vi "Main Low-T Experiments.vi"() -> ()   [LabVIEW 2012]
uses:
  Global Vars.vi
  Channels.vi
  States.ctl
  <vilib>/DAQmx/read.llb/DAQmx Read (Counter U32 1Chan 1Samp).vi
  <vilib>/DAQmx/create/channels.llb/DAQmx Create Channel (CI-Count Edges).vi
  Strict Type Def - Scan Parameters Cluster.ctl
  Rabi Window Parameters.ctl
  ESR Window Parameters.ctl
  Strict Type Def - Optimize Parameters Cluster.ctl
  Spin Echo Window Parameters.ctl
  low-T/Spectrum Window Parameters.ctl
  low-T/Stability Window Parameters.ctl
  Window Parameters-CPMG.ctl
  SaveContrastOptions.ctl
  Window Parameters-XY4.ctl
panel:
  in  "Program":T1(tab)
  in  "Continuous":bool
  in  "Green Laser (low-T)":bool caption="Scan"
  in  "Microwave":bool caption="Scan"
  in  "Green Laser":bool caption="Scan"
  out "Counts Intensity Graph":i32[][](graph)
  in  "Scan Parameters":T2={"X Max"=1.0, "X Min"=-1.0, "X Step"=0.01, "Y Max"=1.5, "Y Min"=-1.5, "Y Step"=0.01, "Dwell Time (ms) "=1} {"Dwell Time (ms)" min=0; "Y Step" min=0.0; "X Step" min=0.0}
  in  "Optimize":bool
  in  "Scan":bool
  in  "Count":bool caption="Optimize"
  out "Counts Chart":u32(graph)
  out "Counts/s":i32
  in  "Optimize Parameters":T3={"Volt Step"={"X"=0.01, "Y"=0.01, "Z"=0.0}, "Num Iterations"=5, "Dwell Time (ms)"=10, "Volts Range"={"X"=0.1, "Y"=0.1, "Z"=0.0}, "Method"={"X"=enum."Max", "Y"=enum."Max"}} {"Volts Range"."Z" min=0.0; "Volts Range"."Y" min=0.0; "Volts Range"."X" min=0.0; "Dwell Time (ms)" min=0; "Num Iterations" min=1 step=1; "Volt Step"."Z" min=0.0; "Volt Step"."Y" min=1e-06; "Volt Step"."X" min=1e-06}
  in  "ESR":bool caption="Scan"
  in  "ESR spectrum spreadsheet":path=path "C:/experiment/data/may_15_2012/SIL1_NV1_pippin_uW_off"
  in  "Save ESR spectrum data":bool
  in  "ESR spectrum graph":path=path "C:/experiment/data/may_15_2012/SIL1_NV1_pippin_uW_off"
  in  "Save ESR spectrum graph":bool
  out "Avg ESR spectrum":cluster{"Y":dbl[], "Y":dbl[]}[](graph)
  out "Counts vs. frequency":i32[][](graph)
  in  "# freq points":i32=61
  in  "MW start freq (GHz)":dbl=2.84
  in  "MW stop freq (GHz)":dbl=2.9
  in  "# scans before track":i32=10
  in  "#scan iterations":i32=5
  in  "ESR Parameters":T4={"Window 1 time (s)"=0.012, "Window 2 time (s)"=5e-06, "Window 3 time (s) "=0.02, "Window 4 time (s)"=5e-07, "Window 4 channels"=[TRUE, FALSE, FALSE, TRUE], "Window 3 channels"=[TRUE, FALSE, TRUE, TRUE], "Window 2 channels"=[TRUE, FALSE, FALSE, TRUE], "Window 1 channels"=[TRUE, TRUE, FALSE, TRUE], "Path to ESR Burner"=path "C:/Users/Loncar/Desktop/ESR VIs - Srujan/Sam Kim/PB/ESRFreq.exe"}
  in  "Save Rabi Contrast Options":T5={"Save contrast graph"=FALSE, "Path for contrast graph"=path "C:/experiment/data/may_15_2012/SIL1_NV1_pippin_uW_off", "Save contrast data"=FALSE, "Path for contrast data"=path "C:/experiment/data/may_15_2012/SIL1_NV1_pippin_uW_off"}
  in  "# scan iterations":i32
  in  "Rabi Parameters":T6={"Window 1 time (s)"=3e-06, "Window 2 time (s)"=5e-06, "Window 3 min time (s) "=0.0, "Window 3 max time (s)"=0.0, "Window 4 time (s)"=7.5e-07, "Window 5 time (s)"=2e-07, "Window 6 time (s)"=3e-06, "Window 7 time (s)"=2e-07, "Window 8 time (s)"=1e-07, "# samples before track"=0, "# time axis points"=0, "Window 1 active channels"=[FALSE, FALSE, FALSE, TRUE], "Window 2 active channels"=[], "Window 3 active channels"=[TRUE], "Window 4 active channels"=[FALSE, FALSE, FALSE, TRUE], "Window 5 active channels "=[FALSE, FALSE, TRUE, TRUE], "Window 6 active channels"=[FALSE, FALSE, FALSE, TRUE], "Window 7 active channels"=[FALSE, FALSE, TRUE, TRUE], "Window 8 active channels"=[], "Path to Rabi Burner"=path "C:/Users/Loncar/Desktop/ESR VIs - Srujan/Sam Kim/PB/RabiBurn.exe"}
  out "Rabi Normalized contrast":cluster{"Y":dbl[], "Y":dbl[]}[](graph)
  out "Reference counts":cluster{"Y":dbl[], "Y":dbl[]}[](graph)
  out "Readout counts":cluster{"Y":dbl[], "Y":dbl[]}[](graph)
  in  "Rabi":bool caption="Scan"
  in  "SpinEcho Save Options":T5={"Save contrast graph"=FALSE, "Path for contrast graph"=path "C:/experiment/data/may_15_2012/SIL1_NV1_pippin_uW_off", "Save contrast data"=FALSE, "Path for contrast data"=path "C:/experiment/data/may_15_2012/SIL1_NV1_pippin_uW_off"}
  in  "# SpinEcho scan iterations":i32=2
  in  "Spin Echo Parameters":T7={"Path to Spin Echo Burner"=path "C:/Users/Loncar/Desktop/ESR VIs - Srujan/Sam Kim/PB/SpinEchoBurn.exe", "Window 1 time (s)"=3e-06, "Window 1 active channels"=[FALSE, FALSE, FALSE, TRUE], "Window 10 time (s)"=3e-06, "Window 10 active channels"=[FALSE, FALSE, FALSE, TRUE], "# samples"=0, "Window 2 time (s)"=5e-06, "Window 2 active channels"=[], "Window 4 min time (s) "=0.0, "Window 4 active channels"=[FALSE], "Window 8 time (s)"=7.5e-07, "Window 8 active channels"=[FALSE, FALSE, FALSE, TRUE], "Window 9 time (s)"=2e-07, "Window 9 active channels "=[FALSE, FALSE, TRUE, TRUE], "# time axis points"=0, "Window 11 time (s)"=2e-07, "Window 11 active channels"=[FALSE, FALSE, TRUE, TRUE], "Window 12 time (s)"=1e-07, "Window 12 active channels"=[], "Window 4 max time (s)"=0.0, "Window 3 time (s)"=5e-06, "Window 5 time (s)"=5e-06, "Window 3 active channels"=[TRUE, FALSE, FALSE, FALSE], "Window 5 active channels"=[TRUE, FALSE, FALSE, FALSE], "Window 7 time (s)"=5e-06, "Window 7 active channels"=[TRUE, FALSE, FALSE, FALSE]}
  out "Spin Echo contrast":cluster{"Y":dbl[], "Y":dbl[]}[](graph)
  out "Spin Echo Reference":cluster{"Y":dbl[], "Y":dbl[]}[](graph)
  out "SpinEcho Readout":cluster{"Y":dbl[], "Y":dbl[]}[](graph)
  in  "Spin Echo":bool caption="Scan"
  in  "Spectrum":bool caption="Scan"
  out "Average counts":picture
  in  "Path for avg spectrum spreadsheet":path=path "C:/experiment/data/may_15_2012/SIL1_NV1_pippin_uW_off"
  in  "Save avg counts data":bool
  in  "Path for avg spectrum graph":path=path "C:/experiment/data/may_15_2012/SIL1_NV1_pippin_uW_off"
  in  "Save avg spectrum graph":bool
  in  "Save 2D counts array":bool
  in  "Path for 2D counts spreadsheet":path=path "C:/experiment/data/may_15_2012/SIL1_NV1_pippin_uW_off"
  in  "Path for intensity graph":path=path "C:/experiment/data/may_15_2012/SIL1_NV1_pippin_uW_off"
  in  "Save intensity graph":bool
  out "Counts vs. laser voltage":u32[][](graph)
  in  "# V steps":dbl
  in  "V max":dbl=0.3
  in  "V min":dbl=-0.3
  in  "# scans before tracking":i32
  in  "# Spectrum Scan Iterations":i32
  in  "Spectrum Parameters":T8={"Window 1 time (s)"=2e-05, "Window 2 time (s)"=1e-06, "Window 3 time (s) "=5e-08, "Window 4 time (s)"=2e-06, "Path to SpectrumBurn"=path "C:/Users/Loncar/Desktop/ESR VIs - Srujan/Sam Kim/PB/ESRFreq.exe", "Window 5 time (s)"=1e-07, "Window 6 time (s)"=5e-08, "Window 1 active channels"=[FALSE, TRUE], "Window 2 active channels"=[], "Window 3 active channels "=[FALSE, FALSE, TRUE], "Window 4 active channels"=[TRUE, FALSE, TRUE], "Window 5 active channels"=[FALSE, FALSE, TRUE], "Window 6 active channels"=[]}
  in  "Stability":bool caption="Scan"
  in  "Num Scan Iterations":i32
  in  "# V steps":dbl
  in  "V max":dbl=0.3
  in  "V min":dbl=-0.3
  in  "# scans before tracking":i32
  in  "Stability Parameters":T9={"Window 1 time (s)"=2e-05, "Window 2 time (s)"=1e-06, "Window 3 time (s) "=5e-08, "Window 4 time (s)"=2e-06, "Window 5 time (s)"=1e-07, "Window 6 time (s)"=5e-08, "Path to StabilityBurn"=path "C:/Users/Loncar/Desktop/ESR VIs - Srujan/Sam Kim/PB/StabilityBurn.exe", "Window 1 active channels"=[FALSE, TRUE], "Window 2 active channels"=[], "Window 3 active channels "=[FALSE, FALSE, TRUE], "Window 4 active channels"=[TRUE, FALSE, TRUE], "Window 5 active channels"=[FALSE, FALSE, TRUE], "Window 6 active channels"=[]}
  out "Counts vs. laser voltage":u32[][](graph)
  in  "Save intensity graph":bool
  in  "Path for intensity graph":path=path "C:/experiment/data/may_15_2012/SIL1_NV1_pippin_uW_off"
  in  "Path for 2D counts spreadsheet":path=path "C:/experiment/data/may_15_2012/SIL1_NV1_pippin_uW_off"
  in  "Save 2D counts array":bool
  in  "Save avg stability graph":bool
  in  "Path for avg stability graph":path=path "C:/experiment/data/may_15_2012/SIL1_NV1_pippin_uW_off"
  in  "Save avg counts data":bool
  in  "Path for avg spectrum spreadsheet":path=path "C:/experiment/data/may_15_2012/SIL1_NV1_pippin_uW_off"
  out "Average counts":picture
  in  "Save CPMG Contrast Options":T5={"Save contrast graph"=FALSE, "Path for contrast graph"=path "C:/experiment/data/may_15_2012/SIL1_NV1_pippin_uW_off", "Save contrast data"=FALSE, "Path for contrast data"=path "C:/experiment/data/may_15_2012/SIL1_NV1_pippin_uW_off"}
  out "CPMG contrast":cluster{"Y":dbl[], "Y":dbl[]}[](graph)
  out "CPMG Reference counts":cluster{"Y":dbl[], "Y":dbl[]}[](graph)
  out "CPMG Readout counts":cluster{"Y":dbl[], "Y":dbl[]}[](graph)
  in  "CPMG":bool caption="Scan"
  in  "# scan iterations":i32
  in  "CPMG Parameters":T10={"Path to CPMG Burner"=path "C:/Users/Loncar/Desktop/ESR VIs - Srujan/Sam Kim/PB/SpinEchoBurn.exe", "Window 1 time (s)"=3e-06, "Window 1 active channels"=[FALSE, FALSE, FALSE, TRUE], "Window 10 time (s)"=3e-06, "Window 10 active channels"=[FALSE, FALSE, FALSE, TRUE], "Window 2 time (s)"=0.0, "Window 2 active channels"=[], "Window 4 min time (s) "=0.0, "Window 4 active channels"=[FALSE], "Window 8 time (s)"=7.5e-07, "Window 8 active channels"=[FALSE, FALSE, FALSE, TRUE], "Window 9 time (s)"=2e-07, "Window 9 active channels "=[FALSE, FALSE, TRUE, TRUE], "# delay time points"=2, "Window 11 time (s)"=0.0, "Window 11 active channels"=[FALSE, FALSE, TRUE, TRUE], "Window 12 time (s)"=1e-07, "Window 12 active channels"=[], "Window 4 max time (s)"=0.0, "Window 3 time (s)"=0.0, "Window 5 time (s)"=5e-06, "Window 3 active channels"=[TRUE, FALSE, FALSE, FALSE], "Window 5 active channels"=[TRUE, FALSE, FALSE, FALSE], "# pi pulses"=1, "# samples before track"=0} {"# pi pulses" min=1; "# delay time points" min=2}
  in  "Save XY-4 Contrast Options":T5={"Save contrast graph"=FALSE, "Path for contrast graph"=path "C:/experiment/data/may_15_2012/SIL1_NV1_pippin_uW_off", "Save contrast data"=FALSE, "Path for contrast data"=path "C:/experiment/data/may_15_2012/SIL1_NV1_pippin_uW_off"}
  out "XY-4 Normalized contrast":cluster{"Y":dbl[], "Y":dbl[]}[](graph)
  out "XY-4 Reference counts":cluster{"Y":dbl[], "Y":dbl[]}[](graph)
  out "XY-4 Readout counts":cluster{"Y":dbl[], "Y":dbl[]}[](graph)
  in  "XY-4":bool caption="Scan"
  in  "# scan iterations":i32
  in  "XY-4 Parameters":T11={"Path to CPMG Burner"=path "C:/Users/Loncar/Desktop/ESR VIs - Srujan/Sam Kim/PB/SpinEchoBurn.exe", "Window 1 time (s)"=3e-06, "Window 1 active channels"=[FALSE, FALSE, FALSE, TRUE], "Window 10 time (s)"=3e-06, "Window 10 active channels"=[FALSE, FALSE, FALSE, TRUE], "Window 2 time (s)"=0.0, "Window 2 active channels"=[], "Window 4 min time (s) "=0.0, "Window 4 active channels"=[FALSE], "Window 8 time (s)"=7.5e-07, "Window 8 active channels"=[FALSE, FALSE, FALSE, TRUE], "Window 9 time (s)"=2e-07, "Window 9 active channels "=[FALSE, FALSE, TRUE, TRUE], "# time points"=2, "Window 11 time (s)"=0.0, "Window 11 active channels"=[FALSE, FALSE, TRUE, TRUE], "Window 12 time (s)"=1e-07, "Window 12 active channels"=[], "Window 4 max time (s)"=0.0, "Window 3 time (s)"=0.0, "Window 5 time (s)"=5e-06, "Window 3 active channels"=[TRUE, FALSE, FALSE, FALSE], "Window 5c active channels"=[TRUE, FALSE, FALSE, FALSE], "# pulse sequences"=1, "# samples before track"=0, "Window 5a active channels"=[TRUE, FALSE, FALSE, FALSE]} {"# pulse sequences" min=1; "# time points" min=2}
  in  "Laser voltage":tag="Dev1/ao2"
  in  "Counter(s)":tag="Dev1/ctr0"
  in  "X AO Channel":tag="Dev1/ao0"
  in  "Y AO Channel":tag="Dev1/ao1"
  in  "Sample clock line":tag="/Dev1/PFI9"
  in  "spinapi.dll":path=path "C:/SpinCore/SpinAPI/dll/spinapi64.dll"
  in  "HoldChannel.exe":path=path "C:/Users/Loncar/Desktop/ESR VIs - Srujan/Sam Kim/PB/HoldChannel.exe"
  # "Default PB connections:\nPB0 - MW switch\nPB3 - Green AOM\nDefault for low-T:\nPB1 - Green AOM"
  # "ESR spectrum measurement"
  # "Default PB connections:\nPB0 - MW switch\nPB1 - MW freq step\nPB2 - Counter sample clk\nPB3 - Green AOM"
  # "Pulse sequence parameters - Window durations and PB channel states"
  # "Green AOM, MW switch are always on!"
  # "(to spreadsheet)"
  # "MW freq step\ndwell time"
  # "MW freq step"
  # "Wait"
  # "Fluorescence\ncounting"
  # "Ctr sample clk"
  # "Wait"
  # "Rabi measurement"
  # "Default PB connections:\nPB0 - MW switch\nPB1 - unused\nPB2 - Counter sample clk\nPB3 - Green AOM"
  # "to spreadsheet"
  # "Initialization"
  # "Green AOM"
  # "Wait"
  # "All off"
  # "MW pulsing"
  # "MW"
  # "Wait"
  # "Green AOM"
  # "Green AOM,\ncounter sample clk"
  # "Readout"
  # "Repump"
  # "Green AOM"
  # "Green AOM,\ncounter sample clk"
  # "Reference"
  # "All off"
  # "Wait (nominal)"
  # "Spin Echo measurement"
  # "Default PB connections:\nPB0 - MW switch\nPB1 - unused\nPB2 - Counter sample clk\nPB3 - Green AOM"
  # "to spreadsheet"
  # "Green AOM"
  # "Initialization"
  # "All off"
  # "Wait"
  # "MW"
  # "MW pulse 1"
  # "All off"
  # "Free precession 1"
  # "max: ~350"
  # "MW pulse 2"
  # "MW"
  # "Free precession 2: Window 6"
  # "MW"
  # "MW pulse 1"
  # "Green AOM"
  # "Wait"
  # "Green AOM,\ncounter sample clk"
  # "Readout"
  # "Green AOM"
  # "Repump"
  # "Green AOM,\ncounter sample clk"
  # "Reference"
  # "Wait (nominal)"
  # "All off"
  # "(single shot) resonance fluorescence spectroscopy"
  # "Default PB connections:\nPB0 - Red AOM\nPB1 - Green AOM\nPB2 - Counter sample clk"
  # "(to spreadsheet)"
  # "(to spreadsheet)"
  # "Laser Set:"
  # "Spectral stability characterization"
  # "Default PB connections:\nPB0 - Red AOM\nPB1 - Green AOM\nPB2 - Counter sample clk"
  # "(to spreadsheet)"
  # "Laser Set:"
  # "(to spreadsheet)"
  # "CPMG measurement"
  # "Default PB connections:\nPB0 - MW switch\nPB1 - MW 90deg phase shifted\nPB2 - Counter sample clk\nPB3 - Green AOM"
  # "to spreadsheet"
  # "Green AOM"
  # "Initialization"
  # "All off"
  # "Wait"
  # "MW pulse 1\n(pi/2)"
  # "MW"
  # "Free precession\n(Tau/2)"
  # "All off"
  # "max: ~350"
  # "MW pulse 2\n(pi90)"
  # "MW90"
  # "Free precession (Tau/2)\nMW pulse 1 (pi/2)"
  # "Window 6 = Window 4\nWindow 7 = Window 3"
  # "All off\nMW"
  # "Green AOM"
  # "Wait for green"
  # "Green AOM,\ncounter sample clk"
  # "Readout"
  # "Green AOM"
  # "Repump"
  # "Green AOM,\ncounter sample clk"
  # "Reference"
  # "Wait (nominal)"
  # "All off"
  # "XY-4 measurement"
  # "Default PB connections:\nPB0 - MW switch\nPB1 - MW 90deg phase shifted\nPB2 - Counter sample clk\nPB3 - Green AOM"
  # "to spreadsheet"
  # "pulse=XYXY"
  # "max: ~350"
  # "x 4=#pi pulses"
  # "Green AOM"
  # "Initialization"
  # "All off"
  # "Wait"
  # "MW pulse 1\n(pi/2)"
  # "MW"
  # "Free precession\n(T/2)"
  # "All off"
  # "MW (X)"
  # "MW pulse 2\n(pi)"
  # "MW90 (Y)"
  # "Pulse Sequence=[T/2-Pi-T-Pi90-T-Pi-T-Pi90-T/2]^N\nMW pulse 1 (pi/2)"
  # "Window 4-5a-g-6\nWindow 7"
  # "Green AOM"
  # "Wait for green"
  # "Green AOM,\ncounter sample clk"
  # "Readout"
  # "Green AOM"
  # "Repump"
  # "Green AOM,\ncounter sample clk"
  # "Reference"
  # "Wait (nominal)"
  # "All off"
  # "TODO:\nHigh priority:\nPause button on pulsed experiments\nShow counts during pulsed experiments\nMore complex pulse sequences (with IQ mixer)\n\nMedium priority:\nLow-T experiments: spectrum, stability\nChanges in Srujan's low-T experiments\n\nLow priority:\nContinuous Scan does not save image\nSave Counts Intensity Graph as image to clipbard\nAllow ESR to stop and save\n    (1. Stop at end of run; 2. Force stop)\nImplement new tracking algorithm for noisy data\n    (Ensemble NV centers)\nAllow stopping in middle of optimize\nAllow count concurrently with optimize/scan(?)"
  # "Author: Samuel Kim"
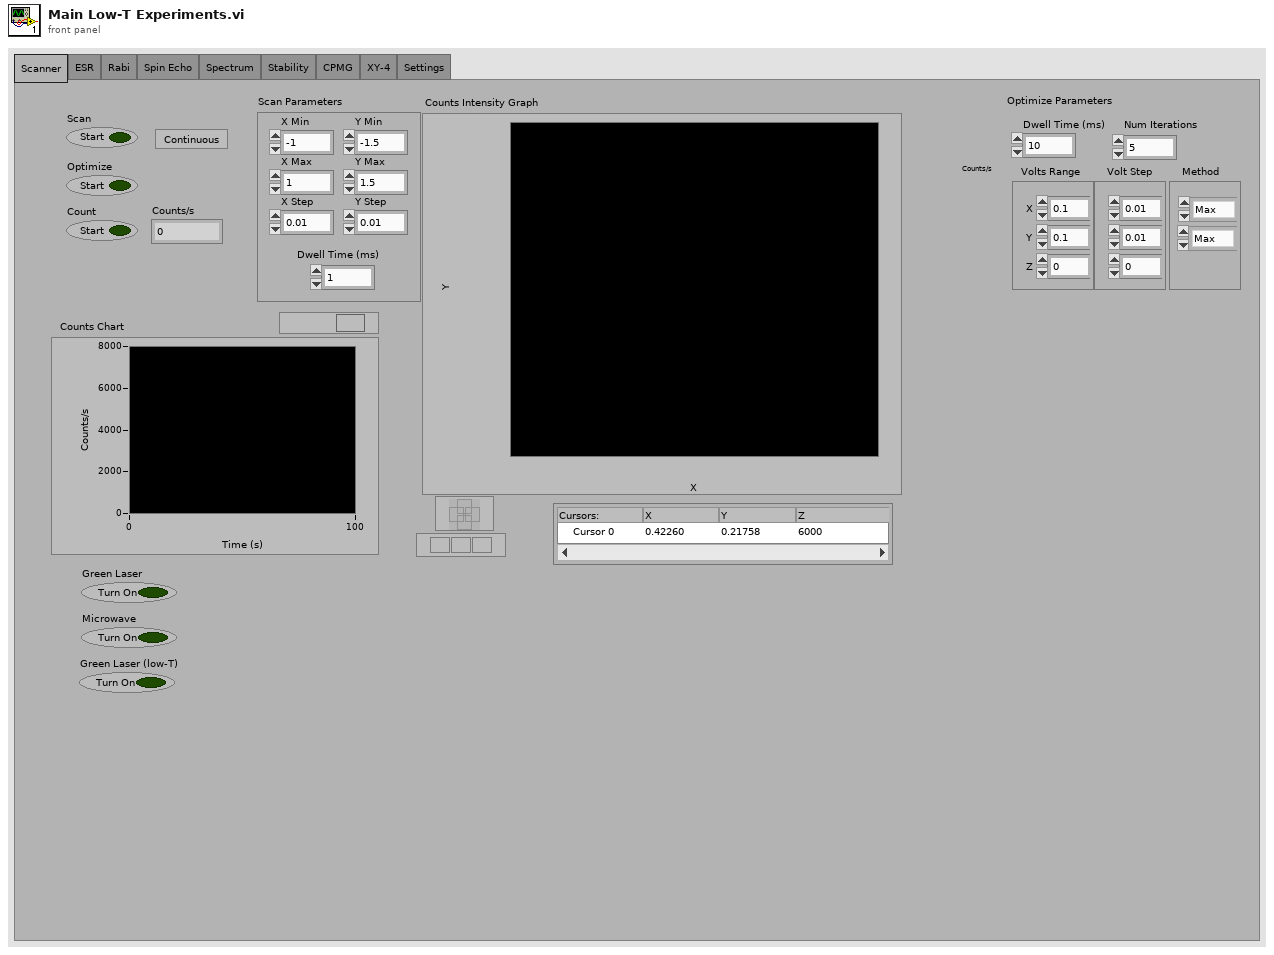
[diagram p1: front panel]
types:
  T1 = enum32{"Scanner", "ESR", "Rabi", "Spin Echo", "Spectrum", "Stability", "CPMG", "XY-4", "Settings"}
  T2 = typedef "Strict Type Def - Scan Parameters Cluster.ctl" = cluster{"X Max":dbl, "X Min":dbl, "X Step":dbl, "Y Max":dbl, "Y Min":dbl, "Y Step":dbl, "Dwell Time (ms) ":i32}
  T3 = typedef "Strict Type Def - Optimize Parameters Cluster.ctl" = cluster{"Volt Step":cluster{"X":dbl, "Y":dbl, "Z":dbl}, "Num Iterations":i32, "Dwell Time (ms)":i32, "Volts Range":cluster{"X":dbl, "Y":dbl, "Z":dbl}, "Method":cluster{"X":enum16{"Max", "Gaussian"}, "Y":enum16{"Max", "Gaussian"}}}
  T4 = typedef "ESR Window Parameters.ctl" = cluster{"Window 1 time (s)":dbl, "Window 2 time (s)":dbl, "Window 3 time (s) ":dbl, "Window 4 time (s)":dbl, "Window 4 channels":bool[], "Window 3 channels":bool[], "Window 2 channels":bool[], "Window 1 channels":bool[], "Path to ESR Burner":path}
  T5 = typedef "SaveContrastOptions.ctl" = cluster{"Save contrast graph":bool, "Path for contrast graph":path, "Save contrast data":bool, "Path for contrast data":path}
  T6 = typedef "Rabi Window Parameters.ctl" = cluster{"Window 1 time (s)":dbl, "Window 2 time (s)":dbl, "Window 3 min time (s) ":dbl, "Window 3 max time (s)":dbl, "Window 4 time (s)":dbl, "Window 5 time (s)":dbl, "Window 6 time (s)":dbl, "Window 7 time (s)":dbl, "Window 8 time (s)":dbl, "# samples before track":i32, "# time axis points":i32, "Window 1 active channels":bool[], "Window 2 active channels":bool[], "Window 3 active channels":bool[], "Window 4 active channels":bool[], "Window 5 active channels ":bool[], "Window 6 active channels":bool[], "Window 7 active channels":bool[], "Window 8 active channels":bool[], "Path to Rabi Burner":path}
  T7 = typedef "Spin Echo Window Parameters.ctl" = cluster{"Path to Spin Echo Burner":path, "Window 1 time (s)":dbl, "Window 1 active channels":bool[], "Window 10 time (s)":dbl, "Window 10 active channels":bool[], "# samples":i32, "Window 2 time (s)":dbl, "Window 2 active channels":bool[], "Window 4 min time (s) ":dbl, "Window 4 active channels":bool[], "Window 8 time (s)":dbl, "Window 8 active channels":bool[], "Window 9 time (s)":dbl, "Window 9 active channels ":bool[], "# time axis points":i32, "Window 11 time (s)":dbl, "Window 11 active channels":bool[], "Window 12 time (s)":dbl, "Window 12 active channels":bool[], "Window 4 max time (s)":dbl, "Window 3 time (s)":dbl, "Window 5 time (s)":dbl, "Window 3 active channels":bool[], "Window 5 active channels":bool[], "Window 7 time (s)":dbl, "Window 7 active channels":bool[]}
  T8 = typedef "Spectrum Window Parameters.ctl" = cluster{"Window 1 time (s)":dbl, "Window 2 time (s)":dbl, "Window 3 time (s) ":dbl, "Window 4 time (s)":dbl, "Path to SpectrumBurn":path, "Window 5 time (s)":dbl, "Window 6 time (s)":dbl, "Window 1 active channels":bool[], "Window 2 active channels":bool[], "Window 3 active channels ":bool[], "Window 4 active channels":bool[], "Window 5 active channels":bool[], "Window 6 active channels":bool[]}
  T9 = typedef "Stability Window Parameters.ctl" = cluster{"Window 1 time (s)":dbl, "Window 2 time (s)":dbl, "Window 3 time (s) ":dbl, "Window 4 time (s)":dbl, "Window 5 time (s)":dbl, "Window 6 time (s)":dbl, "Path to StabilityBurn":path, "Window 1 active channels":bool[], "Window 2 active channels":bool[], "Window 3 active channels ":bool[], "Window 4 active channels":bool[], "Window 5 active channels":bool[], "Window 6 active channels":bool[]}
  T10 = typedef "Window Parameters-CPMG.ctl" = cluster{"Path to CPMG Burner":path, "Window 1 time (s)":dbl, "Window 1 active channels":bool[], "Window 10 time (s)":dbl, "Window 10 active channels":bool[], "Window 2 time (s)":dbl, "Window 2 active channels":bool[], "Window 4 min time (s) ":dbl, "Window 4 active channels":bool[], "Window 8 time (s)":dbl, "Window 8 active channels":bool[], "Window 9 time (s)":dbl, "Window 9 active channels ":bool[], "# delay time points":i32, "Window 11 time (s)":dbl, "Window 11 active channels":bool[], "Window 12 time (s)":dbl, "Window 12 active channels":bool[], "Window 4 max time (s)":dbl, "Window 3 time (s)":dbl, "Window 5 time (s)":dbl, "Window 3 active channels":bool[], "Window 5 active channels":bool[], "# pi pulses":i32, "# samples before track":i32}
  T11 = typedef "Window Parameters-XY4.ctl" = cluster{"Path to CPMG Burner":path, "Window 1 time (s)":dbl, "Window 1 active channels":bool[], "Window 10 time (s)":dbl, "Window 10 active channels":bool[], "Window 2 time (s)":dbl, "Window 2 active channels":bool[], "Window 4 min time (s) ":dbl, "Window 4 active channels":bool[], "Window 8 time (s)":dbl, "Window 8 active channels":bool[], "Window 9 time (s)":dbl, "Window 9 active channels ":bool[], "# time points":i32, "Window 11 time (s)":dbl, "Window 11 active channels":bool[], "Window 12 time (s)":dbl, "Window 12 active channels":bool[], "Window 4 max time (s)":dbl, "Window 3 time (s)":dbl, "Window 5 time (s)":dbl, "Window 3 active channels":bool[], "Window 5c active channels":bool[], "# pulse sequences":i32, "# samples before track":i32, "Window 5a active channels":bool[]}
  T12 = typedef "States.ctl" = enum16{"Initialize", "Scan", "Count", "Optimize", "Hold", "ESR", "Rabi", "Spin Echo", "Spectrum", "Stability", "CPMG", "XY-4", "Exit"}
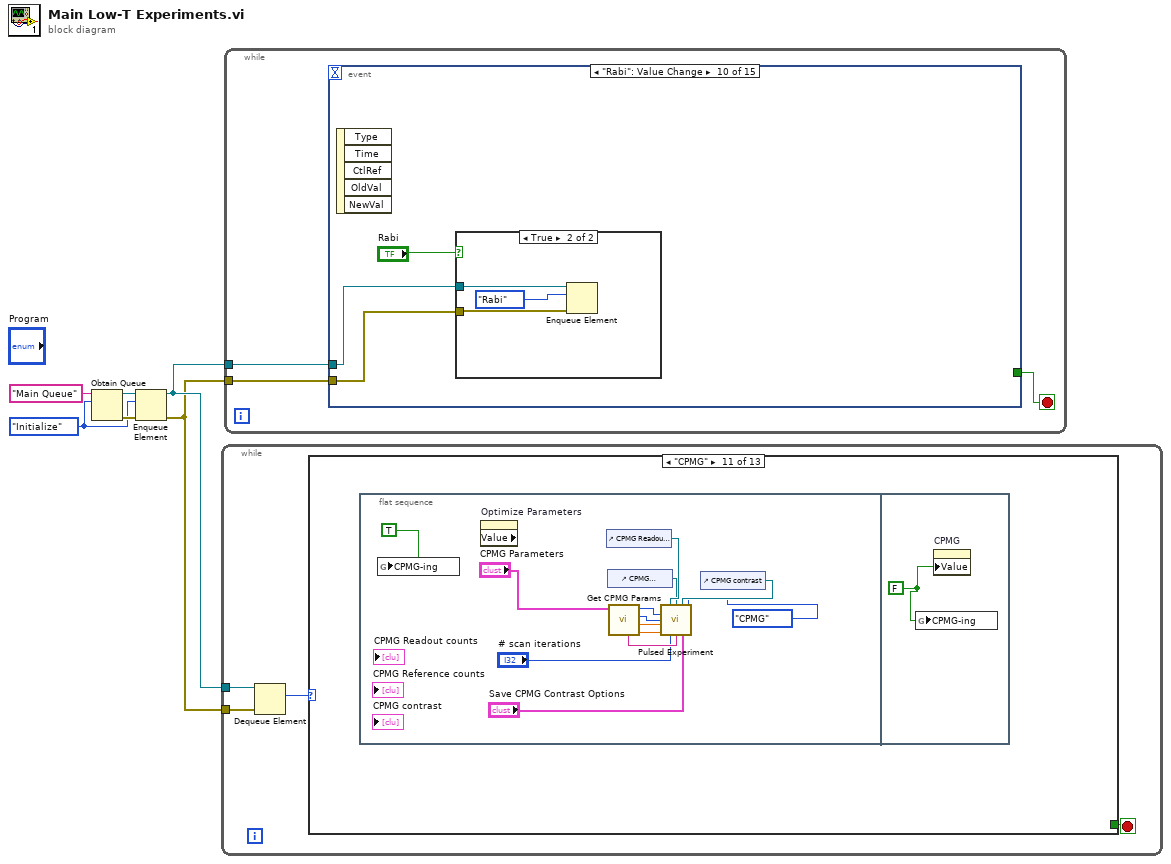
[diagram p0: block diagram]
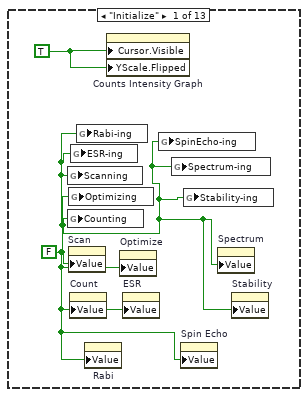
[diagram p2: hidden frame]
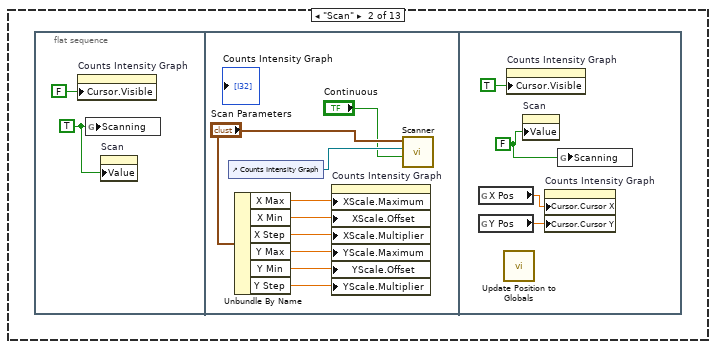
[diagram p3: hidden frame]
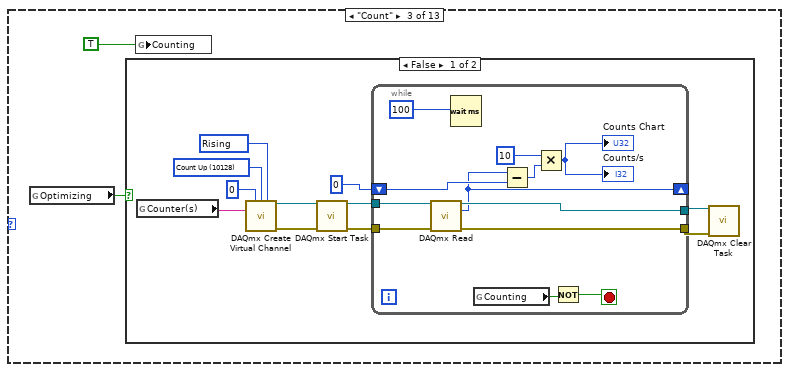
[diagram p4: hidden frame]
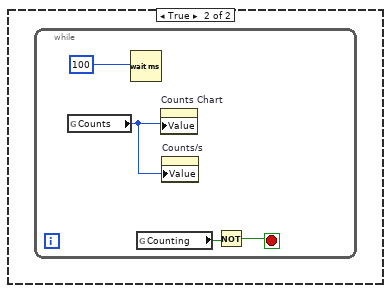
[diagram p5: hidden frame]
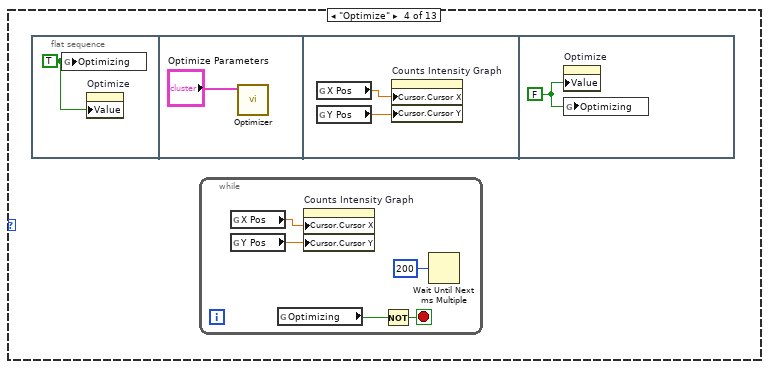
[diagram p6: hidden frame]
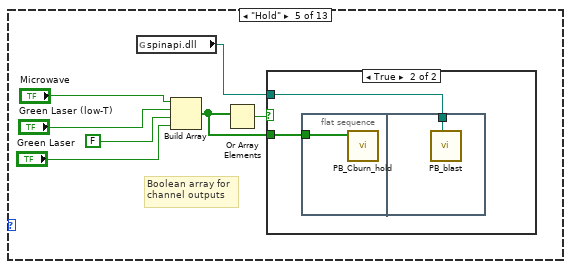
[diagram p7: hidden frame]
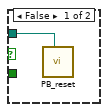
[diagram p8: hidden frame]
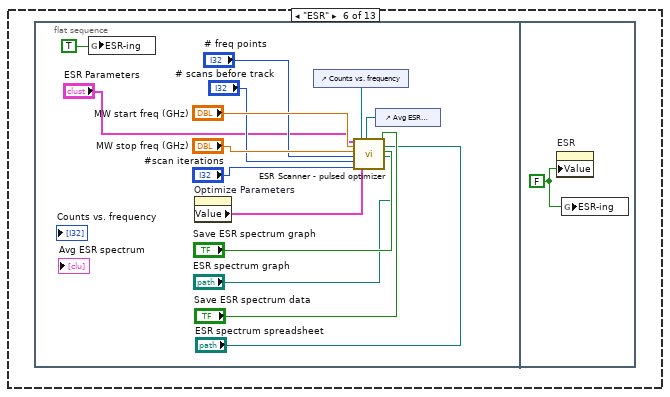
[diagram p9: hidden frame]
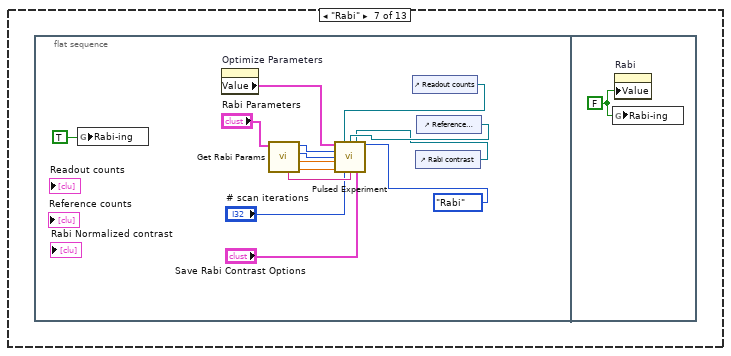
[diagram p10: hidden frame]
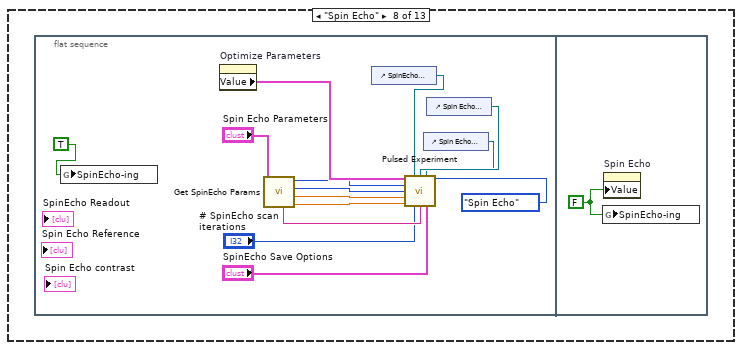
[diagram p11: hidden frame]
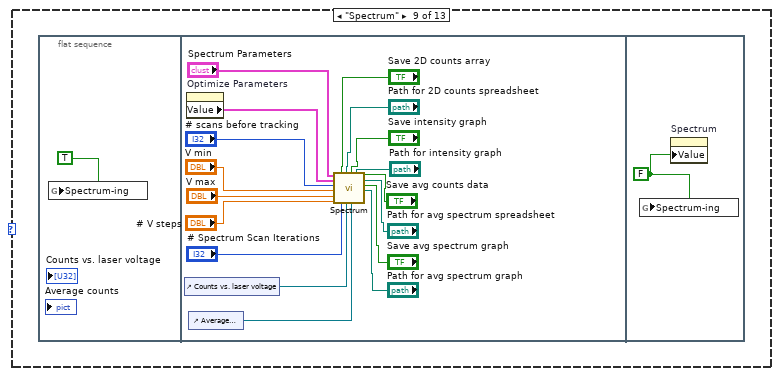
[diagram p12: hidden frame]
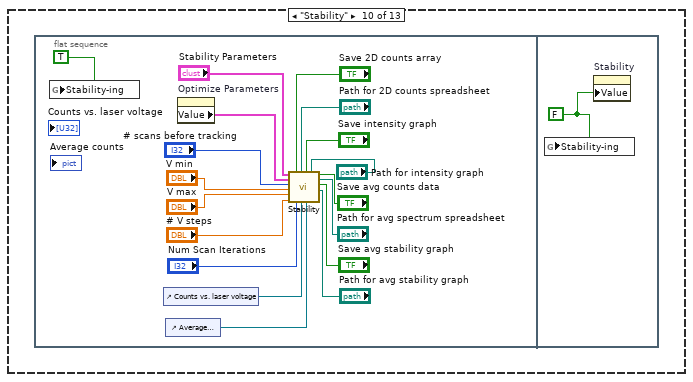
[diagram p13: hidden frame]
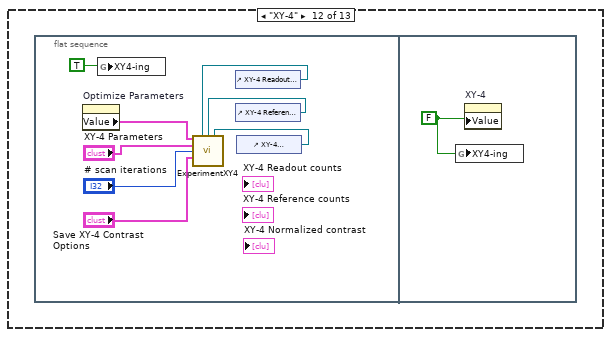
[diagram p14: hidden frame]
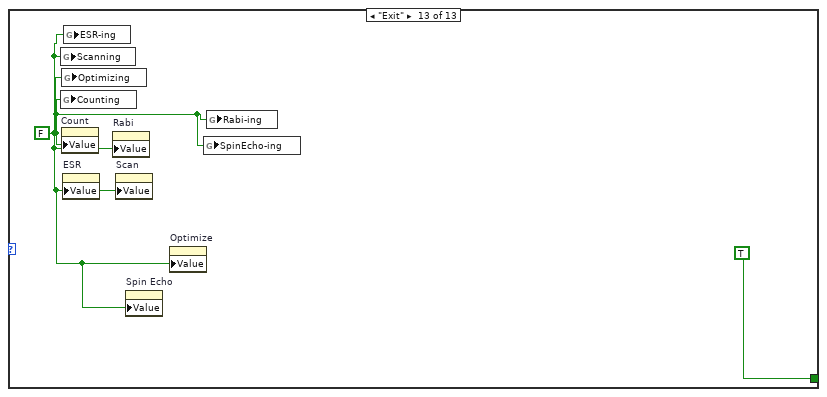
[diagram p15: hidden frame]
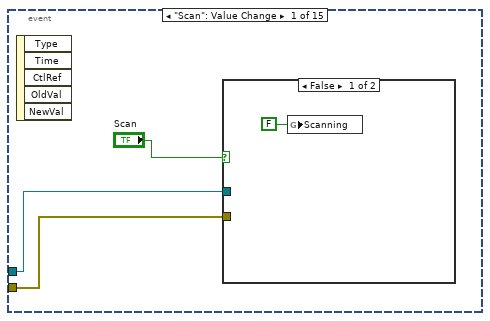
[diagram p16: hidden frame]
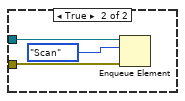
[diagram p17: hidden frame]
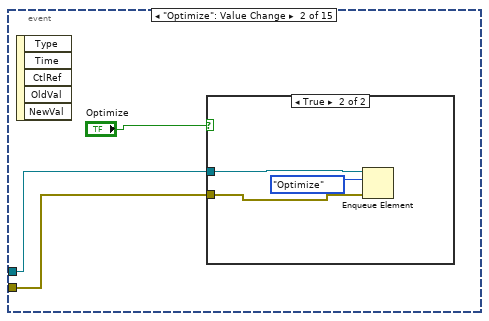
[diagram p18: hidden frame]
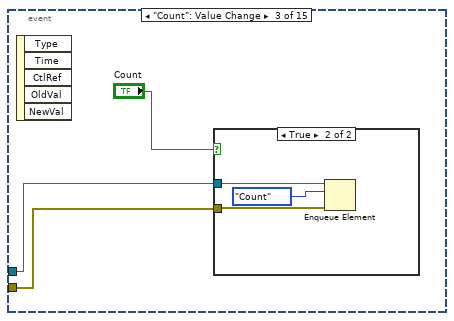
[diagram p20: hidden frame]
diagram:
  w1 = States."Initialize"
  n1 = Obtain Queue(name (unnamed)="Main Queue", element data type=w1) -> (queue out=w4:refnum<queue>, error out=w6:errorcluster)  [unwired: 3 in, 1 out]
  n2 = Enqueue Element(queue=w4, element=w1, error in (no error)=w6) -> (queue out=w3:refnum<queue>, error out=w2:errorcluster)  [unwired: 1 in, 1 out]
  n3 = while {
    tunnel: w3 -> [w9]
    tunnel: w2 -> [w8]
    stop <- w7 stop-if-true
    n4 = Dequeue Element(queue=w9, error in (no error)=w8) -> (element=w10:T12)  [unwired: 1 in, 3 out]
    n5 = case shown="\"CPMG\"" w10 {
      tunnel: [_ _ _ _ _ _ _ _ _ _ _ _ TRUE] -> w7
      frame "Initialize" {
        w12 = TRUE
        w11 = FALSE
        n6 = global write "Global Vars.vi" "Scanning"(w11) -> ()
        n7 = global write "Global Vars.vi" "Counting"(w11) -> ()
        n8 = global write "Global Vars.vi" "Optimizing"(w11) -> ()
        n9 = property on="Scan" class="Bool"("Value"=w11) -> ()  [unwired: 2 in, 2 out]
        n10 = property on="Count" class="Bool (strict)"("Value"=w11) -> ()  [unwired: 2 in, 2 out]
        n11 = global write "Global Vars.vi" "ESR-ing"(w11) -> ()
        n12 = global write "Global Vars.vi" "Rabi-ing"(w11) -> ()
        n13 = property on="Rabi" class="Bool (strict)"("Value"=w11) -> ()  [unwired: 2 in, 2 out]
        n14 = property on="Counts Intensity Graph" class="IntGraph (strict)"("Cursor.Visible"=w12, "YScale.Flipped"=w12) -> ()  [unwired: 2 in, 2 out]
        n15 = property on="Optimize" class="Bool"("Value"=w11) -> ()  [unwired: 2 in, 2 out]
        n16 = property on="ESR" class="Bool (strict)"("Value"=w11) -> ()  [unwired: 2 in, 2 out]
        n17 = global write "Global Vars.vi" "SpinEcho-ing"(w11) -> ()
        n18 = global write "Global Vars.vi" "Spectrum-ing"(w11) -> ()
        n19 = property on="Spin Echo" class="Bool (strict)"("Value"=w11) -> ()  [unwired: 2 in, 2 out]
        n20 = global write "Global Vars.vi" "Stability-ing"(w11) -> ()
        n21 = property on="Spectrum" class="Bool (strict)"("Value"=w11) -> ()  [unwired: 2 in, 2 out]
        n22 = property on="Stability" class="Bool (strict)"("Value"=w11) -> ()  [unwired: 2 in, 2 out]
      }
      frame "Scan" {
        n23 = flat-sequence {
          frame #0 {
            w13 = TRUE
            n24 = property on="Counts Intensity Graph" class="IntGraph (strict)"("Cursor.Visible"=FALSE) -> ()  [unwired: 2 in, 2 out]
            n25 = global write "Global Vars.vi" "Scanning"(w13) -> ()
            n26 = property on="Scan" class="Bool"("Value"=w13) -> ()  [unwired: 2 in, 2 out]
          }
          frame #1 {
            n27 = control-ref of="Counts Intensity Graph"() -> (w23:refnum<vi>)
            n28 = Unbundle By Name("Scan Parameters") -> ("X Max"=w18:dbl, "X Min"=w22:dbl, "X Step"=w21:dbl, "Y Max"=w20:dbl, "Y Min"=w19:dbl, "Y Step"=w16:dbl)
            n29 = property on="Counts Intensity Graph" class="IntGraph (strict)"("XScale.Maximum"=w18, "XScale.Offset"=w22, "XScale.Multiplier"=w21, "YScale.Maximum"=w20, "YScale.Offset"=w19, "YScale.Multiplier"=w16) -> ()  [unwired: 2 in, 2 out]
            n30 = call "Scanner.vi"("Continuous"="Continuous", "IntGraph Refnum"=w23, "Scan Parameters"="Scan Parameters") -> ()  [unwired: 8 in, 1 out]
          }
          frame #2 {
            w24 = FALSE
            n31 = global read "Global Vars.vi" "X Pos"() -> (w26:dbl)
            n32 = global read "Global Vars.vi" "Y Pos"() -> (w25:dbl)
            n33 = call "Update Position to Globals.vi"() -> ()  [unwired: 11 in, 1 out]
            n34 = property on="Counts Intensity Graph" class="IntGraph (strict)"("Cursor.Visible"=TRUE) -> ()  [unwired: 2 in, 2 out]
            n35 = property on="Scan" class="Bool"("Value"=w24) -> ()  [unwired: 2 in, 2 out]
            n36 = property on="Counts Intensity Graph" class="IntGraph (strict)"("Cursor.Cursor X"=w26, "Cursor.Cursor Y"=w25) -> ()  [unwired: 2 in, 2 out]
            n37 = global write "Global Vars.vi" "Scanning"(w24) -> ()
          }
        }
      }
      frame "Count" {
        n38 = global read "Global Vars.vi" "Optimizing"() -> (w28:bool)
        n39 = case shown="False" w28 {
          frame False {
            w38 = 10280 items=["Rising"=10280, "Falling"=10171] ("Edge")
            w39 = 10128 items=["Count Up"=10128, "Count Down"=10124, "Externally Controlled"=10326] ("Count Direction")
            n40 = global read "Channels.vi" "Counter(s)"() -> (w37:tag)
            n41 = call-poly <vilib>:"DAQmx Create Virtual Channel.vi"("initial count"=u32 0 ("Initial Count"), "count direction"=w39, "edge"=w38, "counter"=w37) -> ("task out"=w36:refnum<k21>, "error out"=w35:errorcluster)  [unwired: 10 in]
            n42 = call <vilib>:"DAQmx Start Task.vi"("task/channels in"=w36, "error in"=w35) -> ("task out"=w34:refnum<k21>, "error out"=w33:errorcluster)  [unwired: 12 in]
            n43 = while {
              tunnel: w34 -> [w50]
              tunnel: w33 -> [w49]
              shift-right: [w44] -> _
              shift-left: 0 -> [w48]
              tunnel: [w46] -> w31
              tunnel: [w45] -> w30
              stop <- w51 stop-if-true
              n44 = call-poly <vilib>:"DAQmx Read.vi"("task/channels in"=w50, "error in"=w49) -> ("task out"=w46:refnum<k21>, "data"=w44:u32, "error out"=w45:errorcluster)  [unwired: 11 in]
              n45 = Wait (ms)(milliseconds to wait=100) -> ()  [unwired: 1 out]
              n46 = global read "Global Vars.vi" "Counting"() -> (w52:bool)
              n47 = Subtract(x=w44, y=w48) -> (x-y=w42:u32)
              n48 = Multiply(x=10, y=w42) -> (x*y=→"Counts/s" →"Counts Chart":u32)
              n49 = Not(x=w52) -> (.not. x?=w51:bool)
            }
            n50 = call <vilib>:"DAQmx Clear Task.vi"("task in"=w31, "error in"=w30) -> ()  [unwired: 13 in, 1 out]
          }
          frame True {
            n51 = while {
              stop <- w55 stop-if-true
              n52 = global read "Global Vars.vi" "Counts"() -> (w53:u32)
              n53 = Wait (ms)(milliseconds to wait=100) -> ()  [unwired: 1 out]
              n54 = global read "Global Vars.vi" "Counting"() -> (w56:bool)
              n55 = property on="Counts Chart" class="WFChart (strict)"("Value"=w53) -> ()  [unwired: 2 in, 2 out]
              n56 = property on="Counts/s" class="DigNum (strict)"("Value"=w53) -> ()  [unwired: 2 in, 2 out]
              n57 = Not(x=w56) -> (.not. x?=w55:bool)
            }
          }
        }
        n58 = global write "Global Vars.vi" "Counting"(TRUE) -> ()
      }
      frame "Optimize" {
        n59 = flat-sequence {
          frame #0 {
            w62 = TRUE
            n60 = global write "Global Vars.vi" "Optimizing"(w62) -> ()
            n61 = property on="Optimize" class="Bool"("Value"=w62) -> ()  [unwired: 2 in, 2 out]
          }
          frame #1 {
            n62 = call "Optimizer.vi"("Optimize Parameters"="Optimize Parameters") -> ()  [unwired: 11 in]
          }
          frame #2 {
            n63 = global read "Global Vars.vi" "X Pos"() -> (w65:dbl)
            n64 = global read "Global Vars.vi" "Y Pos"() -> (w64:dbl)
            n65 = property on="Counts Intensity Graph" class="IntGraph (strict)"("Cursor.Cursor X"=w65, "Cursor.Cursor Y"=w64) -> ()  [unwired: 2 in, 2 out]
          }
          frame #3 {
            w66 = FALSE
            n66 = property on="Optimize" class="Bool"("Value"=w66) -> ()  [unwired: 2 in, 2 out]
            n67 = global write "Global Vars.vi" "Optimizing"(w66) -> ()
          }
        }
        n68 = while {
          stop <- w61 stop-if-true
          n69 = global read "Global Vars.vi" "X Pos"() -> (w59:dbl)
          n70 = global read "Global Vars.vi" "Y Pos"() -> (w58:dbl)
          n71 = global read "Global Vars.vi" "Optimizing"() -> (w60:bool)
          n72 = property on="Counts Intensity Graph" class="IntGraph (strict)"("Cursor.Cursor X"=w59, "Cursor.Cursor Y"=w58) -> ()  [unwired: 2 in, 2 out]
          n73 = Not(x=w60) -> (.not. x?=w61:bool)
          n74 = Wait Until Next ms Multiple(millisecond multiple=u32 200) -> ()  [unwired: 1 out]
        }
      }
      frame "Hold" {
        # "Boolean array for\nchannel outputs"
        n75 = global read "Channels.vi" "spinapi.dll"() -> (w73:path)
        n76 = Build Array("Microwave", "Green Laser (low-T)", FALSE, "Green Laser") -> (w67:bool[])
        n77 = Or Array Elements(Boolean array=w67) -> (logical OR=w72:bool)
        n78 = case shown="True" w72 {
          tunnel: w73 -> [w74 w76]
          tunnel: w67 -> [_ w75]
          frame False {
            n79 = call "PB_reset.vi"("Path to spinapi.dll"=w74) -> ()  [unwired: 7 in]
          }
          frame True {
            n80 = flat-sequence {
              tunnel: w75 -> [w77]
              tunnel: w76 -> [w78]
              frame #0 {
                n81 = call "PB_Cburn_hold.vi"("Optimize active channels"=w77) -> ()  [unwired: 9 in, 2 out]
              }
              frame #1 {
                n82 = call "PB_blast.vi"("Path to spinapi.dll"=w78) -> ()  [unwired: 7 in]
              }
            }
          }
        }
      }
      frame "ESR" {
        n83 = flat-sequence {
          frame #0 {
            n84 = global write "Global Vars.vi" "ESR-ing"(TRUE) -> ()
            n85 = property on="Optimize Parameters" class="Clust (strict)"() -> ("Value"=w83:T3)  [unwired: 2 in, 2 out]
            n86 = control-ref of="Counts vs. frequency"() -> (w85:refnum<vi>)
            n87 = control-ref of="Avg ESR spectrum"() -> (w84:refnum<vi>)
            n88 = call "ESR Scanner - pulsed optimizer.vi"("ESR Parameters"="ESR Parameters", "MW start freq (GHz)"="MW start freq (GHz)", "MW stop freq (GHz)"="MW stop freq (GHz)", "# freq points"="# freq points", "# scans before track"="# scans before track", "#scan iterations"="#scan iterations", "IntGraph Refnum"=w85, "Optimize Parameters"=w83, "XY Graph Refnum"=w84, "Save avg spectrum data to spreadsheet?"="Save ESR spectrum data", "Path for avg spectrum spreadsheet"="ESR spectrum spreadsheet", "Save avg spectrum graph?"="Save ESR spectrum graph", "Path for avg spectrum graph"="ESR spectrum graph") -> ()  [unwired: 7 in]
          }
          frame #1 {
            w93 = FALSE
            n89 = property on="ESR" class="Bool (strict)"("Value"=w93) -> ()  [unwired: 2 in, 2 out]
            n90 = global write "Global Vars.vi" "ESR-ing"(w93) -> ()
          }
        }
      }
      frame "Rabi" {
        n91 = flat-sequence {
          frame #0 {
            n92 = global write "Global Vars.vi" "Rabi-ing"(TRUE) -> ()
            n93 = property on="Optimize Parameters" class="Clust (strict)"() -> ("Value"=w100:T3)  [unwired: 2 in, 2 out]
            n94 = call "Get Rabi Params.vi"("Rabi Parameters"="Rabi Parameters") -> ("max time"=w103:dbl, "min time"=w104:dbl, "# time points"=w105:i32, "# samples"=w106:i32, "PB Window Args"=w102:string)  [unwired: 6 in]
            n95 = control-ref of="Readout counts"() -> (w97:refnum<vi>)
            n96 = control-ref of="Rabi contrast"() -> (w95:refnum<vi>)
            n97 = control-ref of="Reference counts"() -> (w96:refnum<vi>)
            n98 = call "Pulsed Experiment.vi"("Optimize Parameters"=w100, "Readout XY Graph Refnum"=w97, "Reference XY Graph Refnum"=w96, "Contrast XY Graph Refnum"=w95, "Experiment"=States."Rabi", "# samples"=w106, "# time points"=w105, "min time"=w104, "max time"=w103, "# scan iterations"="# scan iterations", "Window Parameters"=w102, "Save Contrast Options"="Save Rabi Contrast Options") -> ()  [unwired: 4 in]
          }
          frame #1 {
            w108 = FALSE
            n99 = global write "Global Vars.vi" "Rabi-ing"(w108) -> ()
            n100 = property on="Rabi" class="Bool (strict)"("Value"=w108) -> ()  [unwired: 2 in, 2 out]
          }
        }
      }
      frame "Spin Echo" {
        n101 = flat-sequence {
          frame #0 {
            n102 = global write "Global Vars.vi" "SpinEcho-ing"(TRUE) -> ()
            n103 = property on="Optimize Parameters" class="Clust (strict)"() -> ("Value"=w120:T3)  [unwired: 2 in, 2 out]
            n104 = call "Get SpinEcho Params.vi"("Spin Echo Parameters"="Spin Echo Parameters") -> ("max time"=w116:dbl, "min time"=w117:dbl, "# time points"=w118:i32, "# samples"=w119:i32, "Window Params Args"=w115:string)  [unwired: 6 in]
            n105 = control-ref of="SpinEcho Readout"() -> (w112:refnum<vi>)
            n106 = control-ref of="Spin Echo contrast"() -> (w110:refnum<vi>)
            n107 = control-ref of="Spin Echo Reference"() -> (w111:refnum<vi>)
            n108 = call "Pulsed Experiment.vi"("Optimize Parameters"=w120, "Readout XY Graph Refnum"=w112, "Reference XY Graph Refnum"=w111, "Contrast XY Graph Refnum"=w110, "Experiment"=States."Spin Echo", "# samples"=w119, "# time points"=w118, "min time"=w117, "max time"=w116, "# scan iterations"="# SpinEcho scan iterations", "Window Parameters"=w115, "Save Contrast Options"="SpinEcho Save Options") -> ()  [unwired: 4 in]
          }
          frame #1 {
            w123 = FALSE
            n109 = global write "Global Vars.vi" "SpinEcho-ing"(w123) -> ()
            n110 = property on="Spin Echo" class="Bool (strict)"("Value"=w123) -> ()  [unwired: 2 in, 2 out]
          }
        }
      }
      frame "Spectrum" {
        n111 = flat-sequence {
          frame #0 {
            n112 = global write "Global Vars.vi" "Spectrum-ing"(TRUE) -> ()
          }
          frame #1 {
            n113 = control-ref of="Counts vs. laser voltage"() -> (w134:refnum<vi>)
            n114 = property on="Optimize Parameters" class="Clust (strict)"() -> ("Value"=w140:T3)  [unwired: 2 in, 2 out]
            n115 = control-ref of="Average counts"() -> (w133:refnum<vi>)
            n116 = call "Spectrum.vi"("Spectrum Parameters"="Spectrum Parameters", "Optimize Parameters"=w140, "Num Scan Iterations"="# scans before tracking", "V min"="V min", "V max"="V max", "# V steps"="# V steps", "Save 2D counts array to spreadsheet?"="Save 2D counts array", "# Samples per laser voltage point"="# Spectrum Scan Iterations", "Path for 2D counts spreadsheet"="Path for 2D counts spreadsheet", "Counts vs laser IntGraph Refnum"=w134, "Save intensity graph?"="Save intensity graph", "Pict Refnum"=w133, "Path for intensity graph"="Path for intensity graph", "Save avg counts data to spreadsheet?"="Save avg counts data", "Path for avg spectrum spreadsheet"="Path for avg spectrum spreadsheet", "Save avg spectrum graph?"="Save avg spectrum graph", "Path for avg spectrum graph"="Path for avg spectrum graph") -> ()  [unwired: 3 in]
          }
          frame #2 {
            w142 = FALSE
            n117 = global write "Global Vars.vi" "Spectrum-ing"(w142) -> ()
            n118 = property on="Spectrum" class="Bool (strict)"("Value"=w142) -> ()  [unwired: 2 in, 2 out]
          }
        }
      }
      frame "Stability" {
        n119 = flat-sequence {
          frame #0 {
            n120 = global write "Global Vars.vi" "Stability-ing"(TRUE) -> ()
            n121 = control-ref of="Counts vs. laser voltage"() -> (w144:refnum<vi>)
            n122 = control-ref of="Average counts"() -> (w143:refnum<vi>)
            n123 = property on="Optimize Parameters" class="Clust (strict)"() -> ("Value"=w158:T3)  [unwired: 2 in, 2 out]
            n124 = call "Stability.vi"("Stability Parameters"="Stability Parameters", "Optimize Parameters"=w158, "# Scans"="# scans before tracking", "V min"="V min", "V max"="V max", "# V steps"="# V steps", "Save 2D counts array to spreadsheet"="Save 2D counts array", "Num Scan Iterations"="Num Scan Iterations", "Path for 2D counts spreadsheet"="Path for 2D counts spreadsheet", "Counts vs laser IntGraph Refnum"=w144, "Save intensity graph"="Save intensity graph", "Pict Refnum"=w143, "Path for intensity graph"="Path for intensity graph", "Save avg counts data"="Save avg counts data", "Path for avg spectrum spreadsheet"="Path for avg spectrum spreadsheet", "Save avg spectrum graph?"="Save avg stability graph", "Path for avg spectrum graph"="Path for avg stability graph") -> ()  [unwired: 3 in]
          }
          frame #1 {
            w161 = FALSE
            n125 = global write "Global Vars.vi" "Stability-ing"(w161) -> ()
            n126 = property on="Stability" class="Bool (strict)"("Value"=w161) -> ()  [unwired: 2 in, 2 out]
          }
        }
      }
      frame "CPMG" {
        n127 = flat-sequence {
          frame #0 {
            n128 = global write "Global Vars.vi" "CPMG-ing"(TRUE) -> ()
            n129 = property on="Optimize Parameters" class="Clust (strict)" props=["Value"]() -> ()  [unwired: 2 in, 3 out]
            n130 = control-ref of="CPMG Readout counts"() -> (w165:refnum<vi>)
            n131 = control-ref of="CPMG Reference counts"() -> (w164:refnum<vi>)
            n132 = call "Get CPMG Params.vi"("CPMG Parameters"="CPMG Parameters") -> ("max time"=w173:dbl, "min time"=w172:dbl, "# time points"=w171:i32, "# samples"=w170:i32, "Window Params Args"=w169:string)  [unwired: 6 in]
            n133 = control-ref of="CPMG contrast"() -> (w163:refnum<vi>)
            n134 = call "Pulsed Experiment.vi"("Readout XY Graph Refnum"=w165, "Reference XY Graph Refnum"=w164, "Contrast XY Graph Refnum"=w163, "Experiment"=States."CPMG", "# samples"=w170, "# time points"=w171, "min time"=w172, "max time"=w173, "# scan iterations"="# scan iterations", "Window Parameters"=w169, "Save Contrast Options"="Save CPMG Contrast Options") -> ()  [unwired: 5 in]
          }
          frame #1 {
            w175 = FALSE
            n135 = global write "Global Vars.vi" "CPMG-ing"(w175) -> ()
            n136 = property on="CPMG" class="Bool (strict)"("Value"=w175) -> ()  [unwired: 2 in, 2 out]
          }
        }
      }
      frame "XY-4" {
        n137 = flat-sequence {
          frame #0 {
            n138 = property on="Optimize Parameters" class="Clust (strict)"() -> ("Value"=w183:T3)  [unwired: 2 in, 2 out]
            n139 = global write "Global Vars.vi" "XY4-ing"(TRUE) -> ()
            n140 = control-ref of="XY-4 Readout counts"() -> (w177:refnum<vi>)
            n141 = control-ref of="XY-4 Reference counts"() -> (w178:refnum<vi>)
            n142 = control-ref of="XY-4 Normalized contrast"() -> (w179:refnum<vi>)
            n143 = call "ExperimentXY4.vi"("Optimize Parameters"=w183, "Readout XY Graph Refnum"=w177, "Reference XY Graph Refnum"=w178, "Contrast XY Graph Refnum"=w179, "XY-4 Parameters"="XY-4 Parameters", "# scan iterations"="# scan iterations", "Save Contrast Options"="Save XY-4 Contrast Options") -> ()  [unwired: 9 in]
          }
          frame #1 {
            w184 = FALSE
            n144 = global write "Global Vars.vi" "XY4-ing"(w184) -> ()
            n145 = property on="XY-4" class="Bool (strict)"("Value"=w184) -> ()  [unwired: 2 in, 2 out]
          }
        }
      }
      frame "Exit" {
        w185 = FALSE
        n146 = global write "Global Vars.vi" "Scanning"(w185) -> ()
        n147 = global write "Global Vars.vi" "Counting"(w185) -> ()
        n148 = global write "Global Vars.vi" "Optimizing"(w185) -> ()
        n149 = property on="Count" class="Bool (strict)"("Value"=w185) -> ()  [unwired: 2 in, 2 out]
        n150 = property on="ESR" class="Bool (strict)"("Value"=w185) -> ()  [unwired: 2 in, 2 out]
        n151 = global write "Global Vars.vi" "ESR-ing"(w185) -> ()
        n152 = property on="Rabi" class="Bool (strict)"("Value"=w185) -> ()  [unwired: 2 in, 2 out]
        n153 = property on="Scan" class="Bool"("Value"=w185) -> ()  [unwired: 2 in, 2 out]
        n154 = property on="Spin Echo" class="Bool (strict)"("Value"=w185) -> ()  [unwired: 2 in, 2 out]
        n155 = property on="Optimize" class="Bool"("Value"=w185) -> ()  [unwired: 2 in, 2 out]
        n156 = global write "Global Vars.vi" "SpinEcho-ing"(w185) -> ()
        n157 = global write "Global Vars.vi" "Rabi-ing"(w185) -> ()
      }
    }
  }
  n158 = while {
    tunnel: w3 -> [w189]
    tunnel: w2 -> [w188]
    stop <- w187 stop-if-true
    n159 = event shown="[9] \"Rabi\": Value Change" {
      selector: _ -> [_ _ _ _ _ _ _ _ _ _ _ _ _ _ _]
      dyn-events: _ -> [_ _ _ _ _ _ _ _ _ _ _ _ _ _ _]
      timeout: _ -> [_ _ _ _ _ _ _ _ _ _ _ _ _ _ _]
      tunnel: w189 -> [w191 w198 w205 _ w214 w223 _ _ w233 w237 w244 w252 w259 w265 w273]
      tunnel: w188 -> [w190 w197 w204 _ w215 w222 _ _ w232 w236 w245 w251 w258 w264 w272]
      tunnel: [_ _ _ _ _ _ _ _ TRUE _ _ _ _ _ _] -> w187
      event "Scan": Value Change {
        n160 = event-data() -> ()  [unwired: 1 in, 5 out]
        n161 = case shown="False" "Scan" {
          tunnel: w191 -> [_ w195]
          tunnel: w190 -> [_ w194]
          frame False {
            n162 = global write "Global Vars.vi" "Scanning"(FALSE) -> ()
          }
          frame True {
            n163 = Enqueue Element(queue=w195, element=States."Scan", error in (no error)=w194) -> ()  [unwired: 1 in, 3 out]
          }
        }
      }
      event "Optimize": Value Change {
        n164 = event-data() -> ()  [unwired: 1 in, 5 out]
        n165 = case shown="True" "Optimize" {
          tunnel: w198 -> [_ w201]
          tunnel: w197 -> [_ w200]
          frame False {
          }
          frame True {
            n166 = Enqueue Element(queue=w201, element=States."Optimize", error in (no error)=w200) -> ()  [unwired: 1 in, 3 out]
          }
        }
      }
      event "Count": Value Change {
        n167 = event-data() -> ()  [unwired: 1 in, 5 out]
        n168 = case shown="True" "Count" {
          tunnel: w205 -> [_ w208]
          tunnel: w204 -> [_ w207]
          frame False {
            n169 = global write "Global Vars.vi" "Counting"(FALSE) -> ()
          }
          frame True {
            n170 = Enqueue Element(queue=w208, element=States."Count", error in (no error)=w207) -> ()  [unwired: 1 in, 3 out]
          }
        }
      }
      event "Counts Intensity Graph": Cursor Release {
        n171 = event-data() -> ("CursLoc"=w210:cluster{"X":dbl, "Y":dbl})  [unwired: 1 in, 7 out]
        n172 = flat-sequence {
          tunnel: w210 -> [w211]
          frame #0 {
            n173 = Unbundle By Name(w211) -> ("X"=w213:dbl, "Y"=w212:dbl)
            n174 = global write "Global Vars.vi" "X Pos"(w213) -> ()
            n175 = global write "Global Vars.vi" "Y Pos"(w212) -> ()
          }
          frame #1 {
            n176 = call "Update Position to Globals.vi"() -> ()  [unwired: 11 in, 1 out]
          }
        }
      }
      event "ESR": Value Change {
        n177 = event-data() -> ()  [unwired: 1 in, 5 out]
        n178 = case shown="True" "ESR" {
          tunnel: w214 -> [_ w219]
          tunnel: w215 -> [_ w218]
          frame False {
            n179 = global write "Global Vars.vi" "ESR-ing"(FALSE) -> ()
          }
          frame True {
            n180 = Enqueue Element(queue=w219, element=States."ESR", error in (no error)=w218) -> ()  [unwired: 1 in, 3 out]
          }
        }
      }
      event "Green Laser", "Microwave", "Green Laser (low-T)": Value Change {
        n181 = event-data() -> ()  [unwired: 1 in, 5 out]
        n182 = Enqueue Element(queue=w223, element=States."Hold", error in (no error)=w222) -> ()  [unwired: 1 in, 3 out]
      }
      event Timeout {
        n183 = event-data() -> ()  [unwired: 1 in, 2 out]
      }
      event "X AO Channel", "Y AO Channel", "Counter(s)", "Sample clock line", "spinapi.dll", "HoldChannel.exe", "Laser voltage": Value Change {
        n184 = event-data() -> ()  [unwired: 1 in, 5 out]
        n185 = global write "Channels.vi" "Laser voltage"("Laser voltage") -> ()
        n186 = global write "Channels.vi" "X Channel"("X AO Channel") -> ()
        n187 = global write "Channels.vi" "Y Channel"("Y AO Channel") -> ()
        n188 = global write "Channels.vi" "Counter(s)"("Counter(s)") -> ()
        n189 = global write "Channels.vi" "Sample clock line"("Sample clock line") -> ()
        n190 = global write "Channels.vi" "HoldChannel.exe"("HoldChannel.exe") -> ()
        n191 = global write "Channels.vi" "spinapi.dll"("spinapi.dll") -> ()
      }
      event Panel Close? {
        w231 = FALSE
        n192 = event-data() -> ()  [unwired: 1 in, 3 out]
        n193 = Enqueue Element(queue=w233, element=States."Exit", error in (no error)=w232) -> ()  [unwired: 1 in, 3 out]
        n194 = global write "Global Vars.vi" "Optimizing"(w231) -> ()
        n195 = global write "Global Vars.vi" "Scanning"(w231) -> ()
        n196 = global write "Global Vars.vi" "Counting"(w231) -> ()
        n197 = global write "Global Vars.vi" "ESR-ing"(w231) -> ()
        n198 = event-data() -> ()  [unwired: 2 in, 1 out]
      }
      event "Rabi": Value Change {
        n199 = event-data() -> ()  [unwired: 1 in, 5 out]
        n200 = case shown="True" "Rabi" {
          tunnel: w237 -> [_ w241]
          tunnel: w236 -> [_ w240]
          frame False {
            n201 = global write "Global Vars.vi" "Rabi-ing"(FALSE) -> ()
          }
          frame True {
            n202 = Enqueue Element(queue=w241, element=States."Rabi", error in (no error)=w240) -> ()  [unwired: 1 in, 3 out]
          }
        }
      }
      event "Spin Echo": Value Change {
        n203 = event-data() -> ()  [unwired: 1 in, 5 out]
        n204 = case shown="True" "Spin Echo" {
          tunnel: w244 -> [_ w248]
          tunnel: w245 -> [_ w247]
          frame False {
            n205 = global write "Global Vars.vi" "SpinEcho-ing"(FALSE) -> ()
          }
          frame True {
            n206 = Enqueue Element(queue=w248, element=States."Spin Echo", error in (no error)=w247) -> ()  [unwired: 1 in, 3 out]
          }
        }
      }
      event "Spectrum": Value Change {
        n207 = event-data() -> ()  [unwired: 1 in, 5 out]
        n208 = case shown="False" "Spectrum" {
          tunnel: w252 -> [_ w255]
          tunnel: w251 -> [_ w254]
          frame False {
            n209 = global write "Global Vars.vi" "Spectrum-ing"(FALSE) -> ()
          }
          frame True {
            n210 = Enqueue Element(queue=w255, element=States."Spectrum", error in (no error)=w254) -> ()  [unwired: 1 in, 3 out]
          }
        }
      }
      event "Stability": Value Change {
        n211 = event-data() -> ()  [unwired: 1 in, 5 out]
        n212 = case shown="False" "Stability" {
          tunnel: w259 -> [_ w262]
          tunnel: w258 -> [_ w261]
          frame False {
            n213 = global write "Global Vars.vi" "Stability-ing"(FALSE) -> ()
          }
          frame True {
            n214 = Enqueue Element(queue=w262, element=States."Stability", error in (no error)=w261) -> ()  [unwired: 1 in, 3 out]
          }
        }
      }
      event "CPMG": Value Change {
        n215 = event-data() -> ()  [unwired: 1 in, 5 out]
        n216 = case shown="False" "CPMG" {
          tunnel: w265 -> [_ w269]
          tunnel: w264 -> [_ w268]
          frame False {
            n217 = global write "Global Vars.vi" "CPMG-ing"(FALSE) -> ()
          }
          frame True {
            n218 = Enqueue Element(queue=w269, element=States."CPMG", error in (no error)=w268) -> ()  [unwired: 1 in, 3 out]
          }
        }
      }
      event "XY-4": Value Change {
        n219 = event-data() -> ()  [unwired: 1 in, 5 out]
        n220 = case shown="True" "XY-4" {
          tunnel: w273 -> [_ w276]
          tunnel: w272 -> [_ w275]
          frame False {
            n221 = global write "Global Vars.vi" "XY4-ing"(FALSE) -> ()
          }
          frame True {
            n222 = Enqueue Element(queue=w276, element=States."XY-4", error in (no error)=w275) -> ()  [unwired: 1 in, 3 out]
          }
        }
      }
    }
  }
